vi "close.vi"(8 "error in (no error)":errorcluster, 11 "BK 9202B in":refnum<class "BK 9202B.lvclass">) -> (0 "error out":errorcluster, 3 "BK 9202B out":refnum<class "BK 9202B.lvclass">)   [LabVIEW 2025, in "Power Supply.lvlib" / "BK 9202B.lvclass"]
uses:
  BK 9202B.lvclass
  BK 9202B.lvclass/BK 9202B.ctl
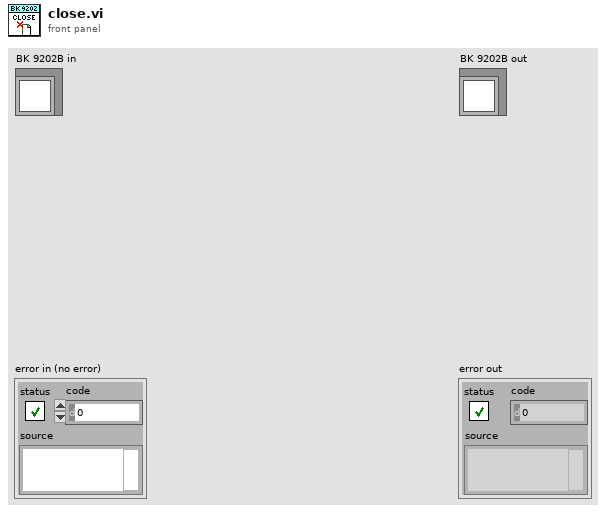
[diagram p1: front panel]
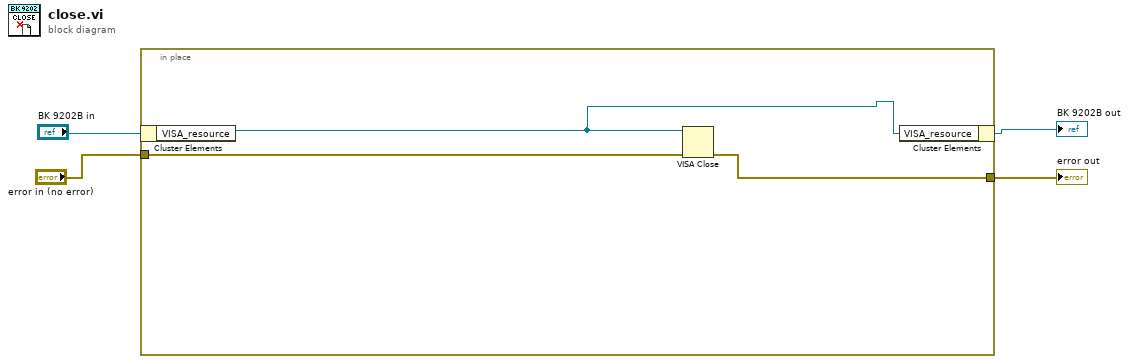
[diagram p0: block diagram]
diagram:
  n1 = in-place {
    in-place-border: "error in (no error)" -> [w6]
    in-place-border: [w5] -> w1
    n2 = in-place-cluster #1("BK 9202B in") -> ("VISA_resource"=w7:refnum<visa-resource-name>)
    n3 = VISA Close(VISA resource name=w7, error in (no error)=w6) -> (error out=w5:errorcluster)
    n4 = in-place-cluster #1("VISA_resource"=w7) -> (→"BK 9202B out":refnum<class "BK 9202B.lvclass">)
  }
  "error out" <- w1
